vi "SUB_COM_WR_Char_timeout.vi"(0 "duplicate VISA resource name":refnum<visa-resource-name>, 1 "cmd string":string, 2 "begin timeTick":u32, 3 "time out seconds":dbl, 4 "Find this String":string) -> (5 "VISA resource OUT":refnum<visa-resource-name>, 6 "Output MSG":string, 7 "Found":bool)   [LabVIEW 2011]
panel:
  out "concatenated string":string
  out "out1":string
  out "LOOP":i32
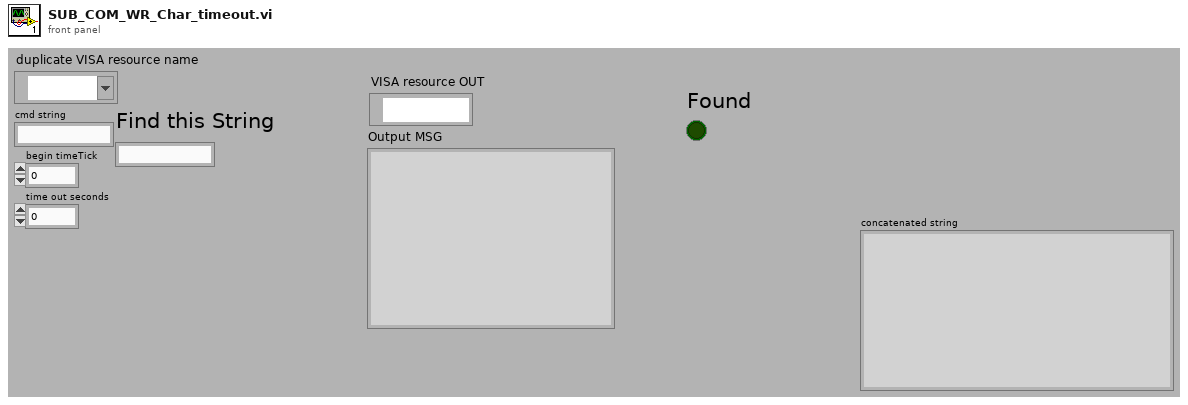
[diagram p1: front panel]
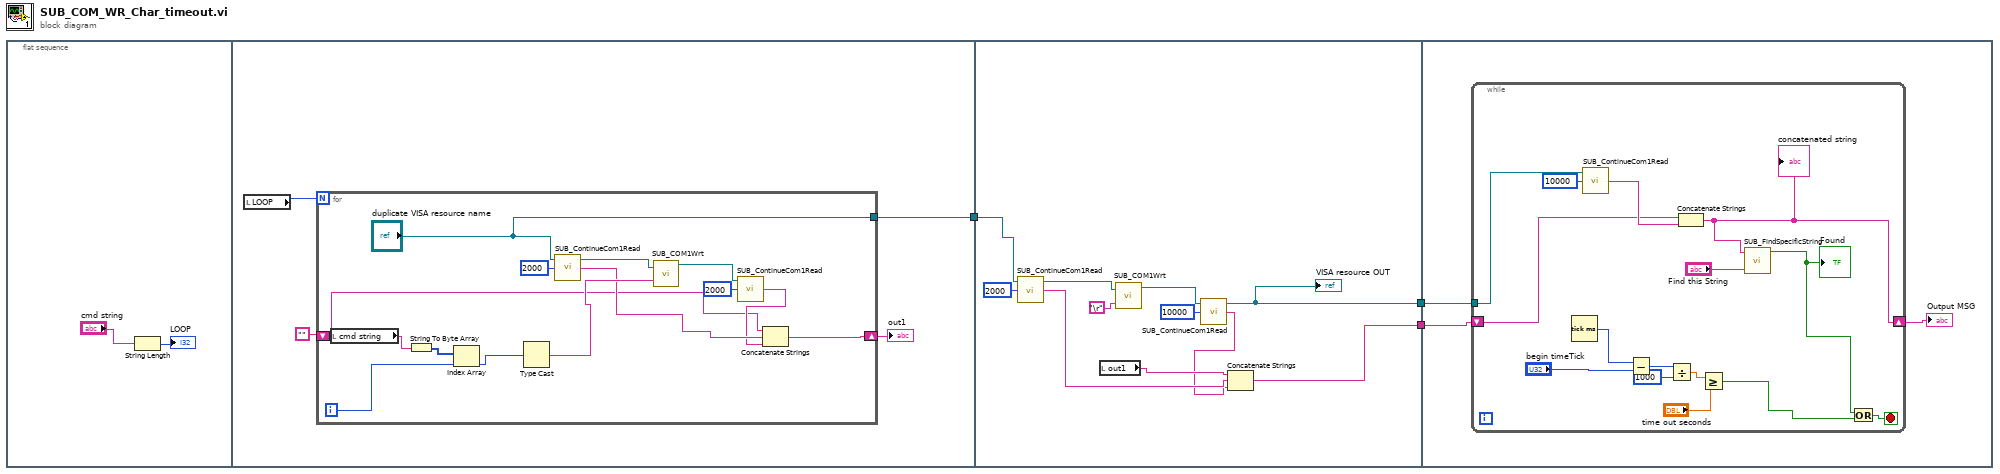
[diagram p0: block diagram]
diagram:
  n1 = flat-sequence {
    tunnel: [w8] -> w3
    tunnel: w3 -> [w26]
    tunnel: [w25] -> w2
    tunnel: [w24] -> w1
    tunnel: w2 -> [w37]
    tunnel: w1 -> [w35]
    frame #0 {
      n2 = String Length(string="cmd string") -> (length=→"LOOP":i32)
    }
    frame #1 {
      n3 = local read "LOOP"() -> (w9:i32)
      n4 = for {
        N: w9 -> [_]
        tunnel: ["duplicate VISA resource name"] -> w8
        shift-right: [w11] -> w6
        shift-left: "" -> [w10]
        i -> [w17]
        n5 = local read "cmd string"() -> (w19:string)
        n6 = String To Byte Array(string=w19) -> (unsigned byte array=w18:u8[])
        n7 = Index Array(array=w18, index=w17) -> (element=w16:u8)
        n8 = Type Cast(x=w16) -> (*(type *) &x=w15:string)  [unwired: 1 in]
        n9 = call "SUB_ContinueCom1Read.vi"("Numeric"=2000, "duplicate VISA resource name 2"="duplicate VISA resource name") -> ("String"=w13:string, "duplicate VISA resource name"=w20:refnum<visa-resource-name>)  [unwired: 1 in, 1 out]
        n10 = call "SUB_COM1Wrt.vi"("VISA resource name"=w20, "write buffer"=w15) -> ("duplicate VISA resource name"=w22:refnum<visa-resource-name>)  [unwired: 2 out]
        n11 = call "SUB_ContinueCom1Read.vi"("Numeric"=2000, "duplicate VISA resource name 2"=w22) -> ("String"=w12:string)  [unwired: 1 in, 2 out]
        n12 = Concatenate Strings(w10, w13, w12) -> (w11:string)
      }
      "out1" <- w6
    }
    frame #2 {
      n13 = call "SUB_ContinueCom1Read.vi"("Numeric"=2000, "duplicate VISA resource name 2"=w26) -> ("String"=w28:string, "duplicate VISA resource name"=w31:refnum<visa-resource-name>)  [unwired: 1 in, 1 out]
      n14 = local read "out1"() -> (w29:string)
      n15 = call "SUB_COM1Wrt.vi"("VISA resource name"=w31, "write buffer"="\r") -> ("duplicate VISA resource name"=w33:refnum<visa-resource-name>)  [unwired: 2 out]
      n16 = call "SUB_ContinueCom1Read.vi"("Numeric"=10000, "duplicate VISA resource name 2"=w33) -> ("String"=w27:string, "duplicate VISA resource name"=w24:refnum<visa-resource-name>)  [unwired: 1 in, 1 out]
      "VISA resource OUT" <- w24
      n17 = Concatenate Strings(w29, w28, w27) -> (w25:string)
    }
    frame #3 {
      n18 = while {
        shift-right: [w50] -> w36
        shift-left: w37 -> [w51]
        tunnel: w35 -> [w39]
        stop <- w48 stop-if-true
        n19 = Tick Count (ms)() -> (millisecond timer value=w46:u32)
        n20 = call "SUB_ContinueCom1Read.vi"("Numeric"=10000, "duplicate VISA resource name 2"=w39) -> ("String"=w52:string)  [unwired: 1 in, 2 out]
        n21 = Subtract(x=w46, y="begin timeTick") -> (x-y=w44:u32)
        n22 = Divide(x=w44, y=u32 1000) -> (x/y=w42:dbl)
        n23 = Concatenate Strings(w51, w52) -> (w50:string)
        "concatenated string" <- w50
        n24 = Greater Or Equal?(x=w42, y="time out seconds") -> (x >= y?=w40:bool)
        n25 = call "SUB_FindSpecificString.vi"("Find this String"="Find this String", "String data"=w50) -> ("Found"=w47:bool)  [unwired: 2 in, 1 out]
        "Found" <- w47
        n26 = Or(x=w47, y=w40) -> (x .or. y?=w48:bool)
      }
      "Output MSG" <- w36
    }
  }
